vi "getChannelList.vi"(4 "error in (no error)":errorcluster, 5 "channel names":string, 6 "group name":string, 7 "TDMS descriptor array":T1(array[cluster])) -> (0 "error out":errorcluster, 1 "channel names out":string[](array[string]), 2 "group names out":string[](array[string]), 3 "TDMS descriptor array out":T1(array[cluster]))   [LabVIEW 2015]
panel:
  in  "tdms file":refnum<k34>
  out "tdms file out":refnum<k34>
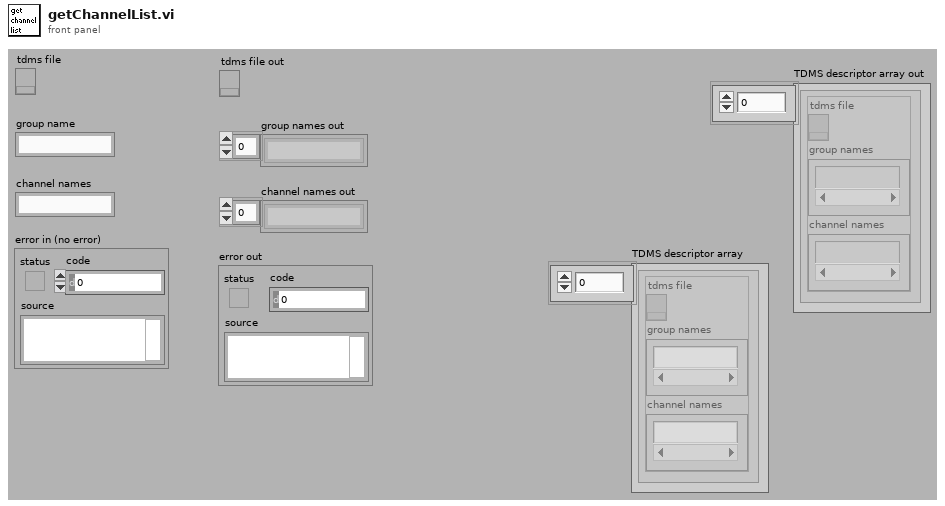
[diagram p1: front panel]
types:
  T1 = cluster{"tdms file ":refnum<k34>, "group names":string[], "channel names":string[]}[]
  T2 = cluster{"tdms file ":refnum<k34>, "group names":string[], "channel names":string[]}
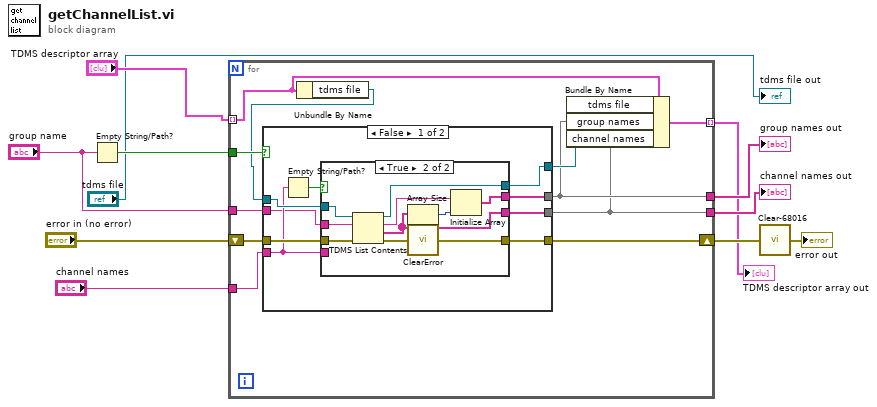
[diagram p0: block diagram]
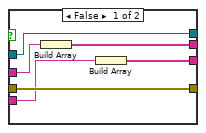
[diagram p2: hidden frame]
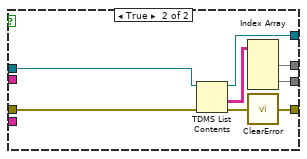
[diagram p3: hidden frame]
diagram:
  n1 = Empty String/Path?(string/path="group name") -> (empty?=w9:bool)
  n2 = for {
    tunnel: [w14] -> w11
    tunnel: "group name" -> [w22]
    tunnel: w9 -> [w21]
    tunnel: [w13] -> w8
    tunnel: "channel names" -> [w20]
    shift-right: [w18] -> w5
    shift-left: "error in (no error)" -> [w19]
    tunnel: "TDMS descriptor array" -> [w16] mode=indexing
    tunnel: [w12] -> w2 mode=indexing
    n3 = Unbundle By Name(w16) -> ("tdms file"=w17:refnum<k34>)
    n4 = case shown="False" w21 {
      tunnel: w17 -> [w30 w55]
      tunnel: w19 -> [w29 w54]
      tunnel: w20 -> [w28 _]
      tunnel: [w27 w52] -> w18
      tunnel: [w26 w53] -> w15
      tunnel: [w25 w51] -> w13
      tunnel: w22 -> [w24 _]
      tunnel: [w23 w50] -> w14
      frame False {
        n5 = Empty String/Path?(string/path=w28) -> (empty?=w31:bool)
        n6 = case shown="True" w31 {
          tunnel: w30 -> [w36 w47]
          tunnel: w29 -> [w37 w46]
          tunnel: [w37 w45] -> w27
          tunnel: [w36 w44] -> w26
          tunnel: w24 -> [w33 w43]
          tunnel: [w34 w39] -> w25
          tunnel: w28 -> [w35 _]
          tunnel: [w32 w40] -> w23
          frame False {
            n7 = Build Array(w33) -> (w32:string[])
            n8 = Build Array(w35) -> (w34:string[])
          }
          frame True {
            n9 = TDMS List Contents(4:w46, 6:w43, 7:w47) -> (0:w38:errorcluster, 1:w39:string[], 2:w41:string, 3:w44:refnum<k34>)
            n10 = Array Size(array=w39) -> (size(s)=w42:i32)
            n11 = call <vilib>:"ClearError.vi"("error in (no error)"=w38) -> ("error out"=w45:errorcluster)
            n12 = Initialize Array(w41, w42) -> (w40:string[])
          }
        }
      }
      frame True {
        n13 = TDMS List Contents(4:w54, 7:w55) -> (0:w48:errorcluster, 1:w49:string[][], 3:w53:refnum<k34>)  [unwired: 1 in, 1 out]
        n14 = Index Array(array=w49) -> (element #1=w50:string[], element #2=w51:string[])  [unwired: 4 in]
        n15 = call <vilib>:"ClearError.vi"("error in (no error)"=w48) -> ("error out"=w52:errorcluster)
      }
    }
    n16 = Bundle By Name(cluster=w16, "tdms file"=w15, "group names"=w14, "channel names"=w13) -> (w12:T2)
  }
  "group names out" <- w11
  "channel names out" <- w8
  "TDMS descriptor array out" <- w2
  n17 = call <vilib>:"Clear-68016.vi"("error in (no error)"=w5) -> ("error out"=→"error out":errorcluster)
  "tdms file out" <- "tdms file"
